vi "Min_size_Template.vi"() -> ()   [LabVIEW 2018]
panel:
  out "Array_Out":variant[](array[variant])
  in  "Size":i32
  in  "Array_In":variant[](array[variant])
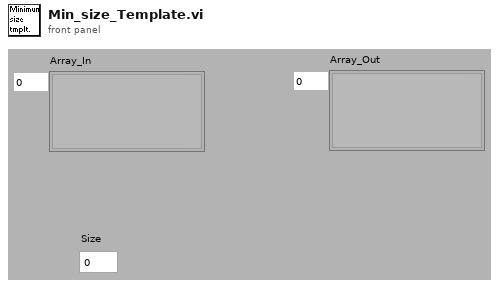
[diagram p1: front panel]
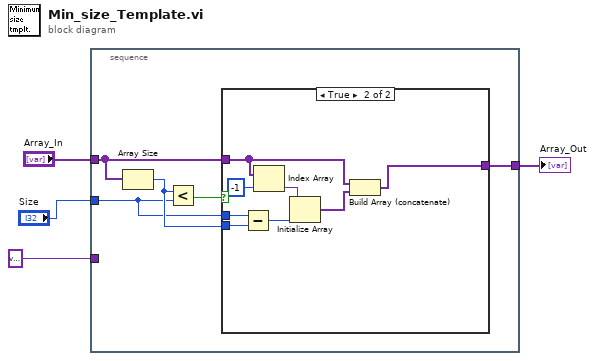
[diagram p0: block diagram]
diagram:
  n1 = stacked-sequence {
    tunnel: "Array_In" -> [w6]
    tunnel: "Size" -> [w7]
    tunnel: variant ("Variant") -> [_]
    tunnel: [w5] -> w1
    frame #0 {
      n2 = Array Size(array=w6) -> (size(s)=w8:i32)
      n3 = Less?(x=w8, y=w7) -> (x < y?=w9:bool)
      n4 = case shown="True" w9 {
        tunnel: w8 -> [_ w18]
        tunnel: w7 -> [_ w17]
        tunnel: w6 -> [w10 w13]
        tunnel: [w10 w15] -> w5
        frame False {
        }
        frame True {
          n5 = Subtract(x=w17, y=w18) -> (x-y=w14:i32)
          n6 = Index Array(array=w13, index=-1) -> (element=w11:variant)
          n7 = Initialize Array(w11, w14) -> (w16:variant[])
          n8 = Build Array (concatenate)(w13, w16) -> (w15:variant[])
        }
      }
    }
  }
  "Array_Out" <- w1
